vi "Storage Control.vi"(3 "Snapshot":T1={"Test Details"="test", "Version"="test", "Date"=timestamp(3493915594.3018084 s since 1904-01-01), "Selected Test"="man", "Snapshot Number"=0, "Time"=timestamp(3493915602.7292905 s since 1904-01-01), "Ibrake Setpoint"="1", "RPM Setpoint"="20", "Range Setpoint"="", "Step Height Setpoint"="", "Load Bank Setpoint"="15", "Measurement Headers"="a,b,c,1,2,3", "Measurements"="1,2,3,4,5,6,7,8", "A"=0, "B"=0, "C"=0, "Raw Data"=[], "Available Tests"=enum."Manual", "Ibrake List"="", "RPM List"="", "Load Bank List"="", "Range List"="", "Step Height List"="", "FanMode Setpoint"=enum."Auto"} {"Time" format="%<%H:%M:%S>T"; "Date" format="%<%m/%d/%Y>T"}, 4 "RPM":dbl, 5 "Torque":dbl, 6 "Snapshot":bool, 7 "Queue Array":T4, 8 "error in (no error)":errorcluster, 9 "Manual Snapshot":bool, 10 "task in":refnum<k21>, 11 "MulticolumnListbox in":refnum<vi>) -> (0 "error out":errorcluster)   [LabVIEW 2017]
uses:
  Code Library/Queue References Array.ctl
  Code Library/Queue Element.ctl
  Controls/Snapshot Typedef.ctl
  Controls/Available Tests.ctl
  Controls/FanMode.ctl
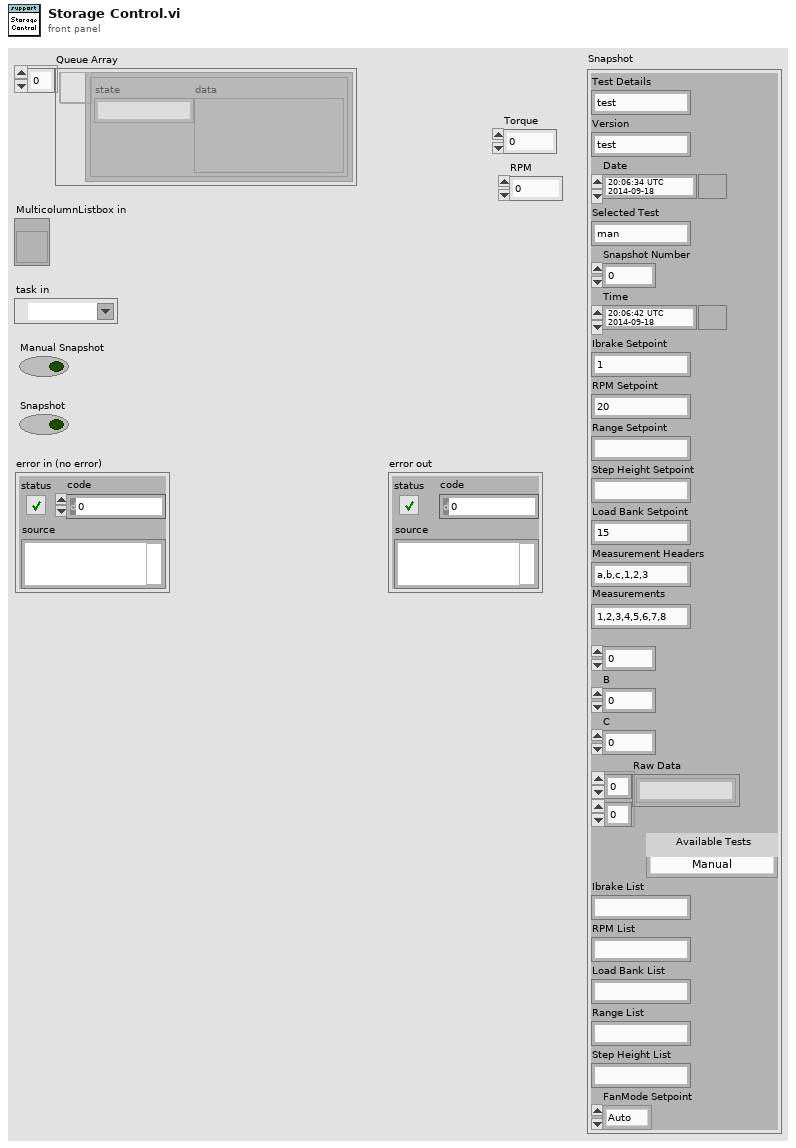
[diagram p1: front panel]
types:
  T1 = typedef "Snapshot Typedef.ctl" = cluster{"Test Details":string, "Version":string, "Date":timestamp, "Selected Test":string, "Snapshot Number":u16, "Time":timestamp, "Ibrake Setpoint":string, "RPM Setpoint":string, "Range Setpoint":string, "Step Height Setpoint":string, "Load Bank Setpoint":string, "Measurement Headers":string, "Measurements":string, "A":i32, "B":i32, "C":i32, "Raw Data":string[][], "Available Tests":T2, "Ibrake List":string, "RPM List":string, "Load Bank List":string, "Range List":string, "Step Height List":string, "FanMode Setpoint":T3}
  T2 = typedef "Available Tests.ctl" = enum16{"Manual", "EFX Brake Torque", "Generator Torque", "EFX Brake Thermal", "Generator Thermal", "Pulsed RPM", "AMT Brake Torque", "Bike Brake Torque", "AMT Brake Thermal", "Bike Brake Thermal"}
  T3 = typedef "FanMode.ctl" = enum16{"On", "Off", "Auto"}
  T4 = typedef "Queue References Array.ctl" = refnum<queue>[]
  T5 = typedef "Queue Element.ctl" = cluster{"state":string, "data":variant}
  T6 = cluster{"task in":refnum<k21>, "MulticolumnListbox in":refnum<vi>, "Snapshot":T1, bool, "Torque":dbl, "RPM":dbl}
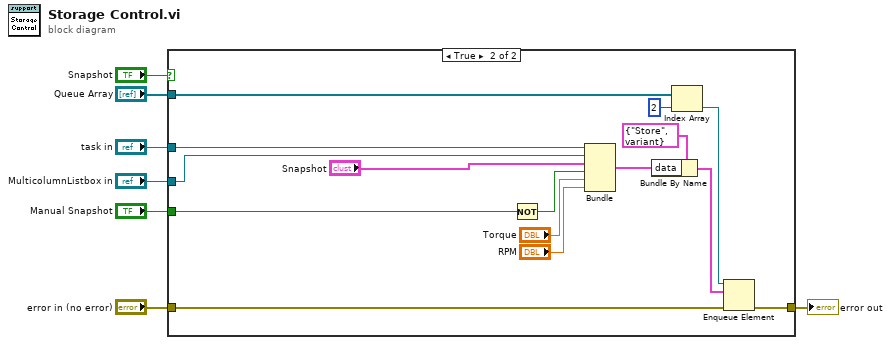
[diagram p0: block diagram]
diagram:
  n1 = case shown="True" "Snapshot" {
    tunnel: "task in" -> [_ w21]
    tunnel: "MulticolumnListbox in" -> [_ w20]
    tunnel: [w8 w23] -> w3
    tunnel: "error in (no error)" -> [w8 w22]
    tunnel: "Queue Array" -> [_ w18]
    tunnel: "Manual Snapshot" -> [_ w12]
    frame False {
    }
    frame True {
      n2 = Not(x=w12) -> (.not. x?=w11:bool)
      n3 = Bundle("task in"=w21, "MulticolumnListbox in"=w20, "Snapshot"="Snapshot", w11, "Torque"="Torque", "RPM"="RPM") -> (w13:T6)  [unwired: 1 in]
      n4 = Bundle By Name(cluster=T5 {"state"="Store", "data"=variant} ("element"), "data"=w13) -> (w14:T5)
      n5 = Index Array(array=w18, index=2) -> (element=w16:refnum<queue>)
      n6 = Enqueue Element(queue=w16, element=w14, error in (no error)=w22) -> (error out=w23:errorcluster)  [unwired: 1 in, 2 out]
    }
  }
  "error out" <- w3
